vi "Lip_Symmetry_new.vi"(0 "Image in":T3(plugin-control), 1 "Lip Outer Perpendicular lines":T2(array[cluster]), 2 "Box Edge Information":T1, 5 "error in (no error)":errorcluster, 6 "Calibrated Image":T3) -> (14 "Lip symmetry":dbl, 19 "error out":errorcluster)   [LabVIEW 2019, in "Algorithm.lvclass"]
uses:
  FrameworkOverrides/Algorithm.lvclass
  <vilib>/vision/NI_Vision_Development_Module.lvlib
  <vilib>/vision/Image Controls.llb/IMAQ Image.ctl
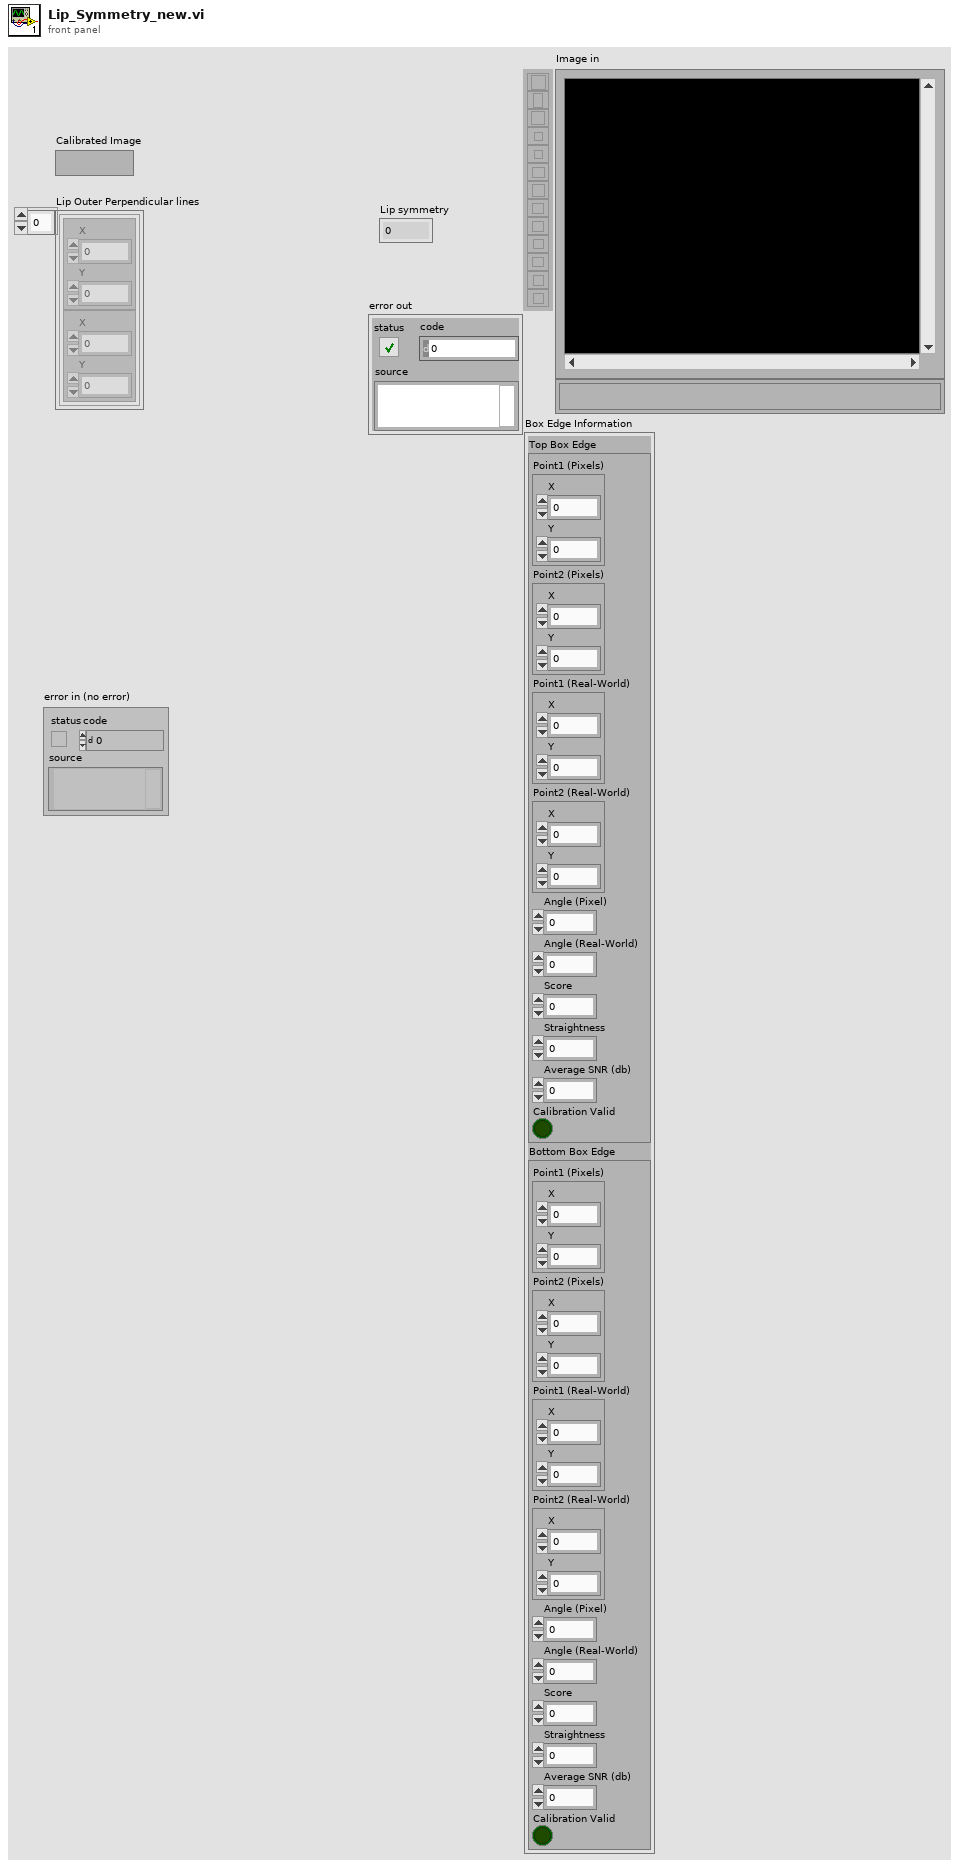
[diagram p1: front panel]
types:
  T1 = cluster{"Top Box Edge":cluster{"Point1 (Pixels)":cluster{"X":sgl, "Y":sgl}, "Point2 (Pixels)":cluster{"X":sgl, "Y":sgl}, "Point1 (Real-World)":cluster{"X":sgl, "Y":sgl}, "Point2 (Real-World)":cluster{"X":sgl, "Y":sgl}, "Angle (Pixel)":dbl, "Angle (Real-World)":dbl, "Score":dbl, "Straightness":dbl, "Average SNR (db)":dbl, "Calibration Valid":bool}, "Bottom Box Edge":cluster{"Point1 (Pixels)":cluster{"X":sgl, "Y":sgl}, "Point2 (Pixels)":cluster{"X":sgl, "Y":sgl}, "Point1 (Real-World)":cluster{"X":sgl, "Y":sgl}, "Point2 (Real-World)":cluster{"X":sgl, "Y":sgl}, "Angle (Pixel)":dbl, "Angle (Real-World)":dbl, "Score":dbl, "Straightness":dbl, "Average SNR (db)":dbl, "Calibration Valid":bool}}
  T2 = cluster{cluster{"X":sgl, "Y":sgl}, cluster{"X":sgl, "Y":sgl}}[]
  T3 = typedef "IMAQ Image.ctl" = refnum<image>
  T4 = cluster{"Point1 (Pixels)":cluster{"X":sgl, "Y":sgl}, "Point2 (Pixels)":cluster{"X":sgl, "Y":sgl}, "Point1 (Real-World)":cluster{"X":sgl, "Y":sgl}, "Point2 (Real-World)":cluster{"X":sgl, "Y":sgl}, "Angle (Pixel)":dbl, "Angle (Real-World)":dbl, "Score":dbl, "Straightness":dbl, "Average SNR (db)":dbl, "Calibration Valid":bool}
  T5 = cluster{"Point1 (Pixels)":cluster{"X":sgl, "Y":sgl}, "Point2 (Pixels)":cluster{"X":sgl, "Y":sgl}}
  T6 = cluster{cluster{"X":sgl, "Y":sgl}, cluster{"X":sgl, "Y":sgl}}
  T7 = cluster{"Point 1":cluster{"X":sgl, "Y":sgl}, "Point 2":cluster{"X":sgl, "Y":sgl}}
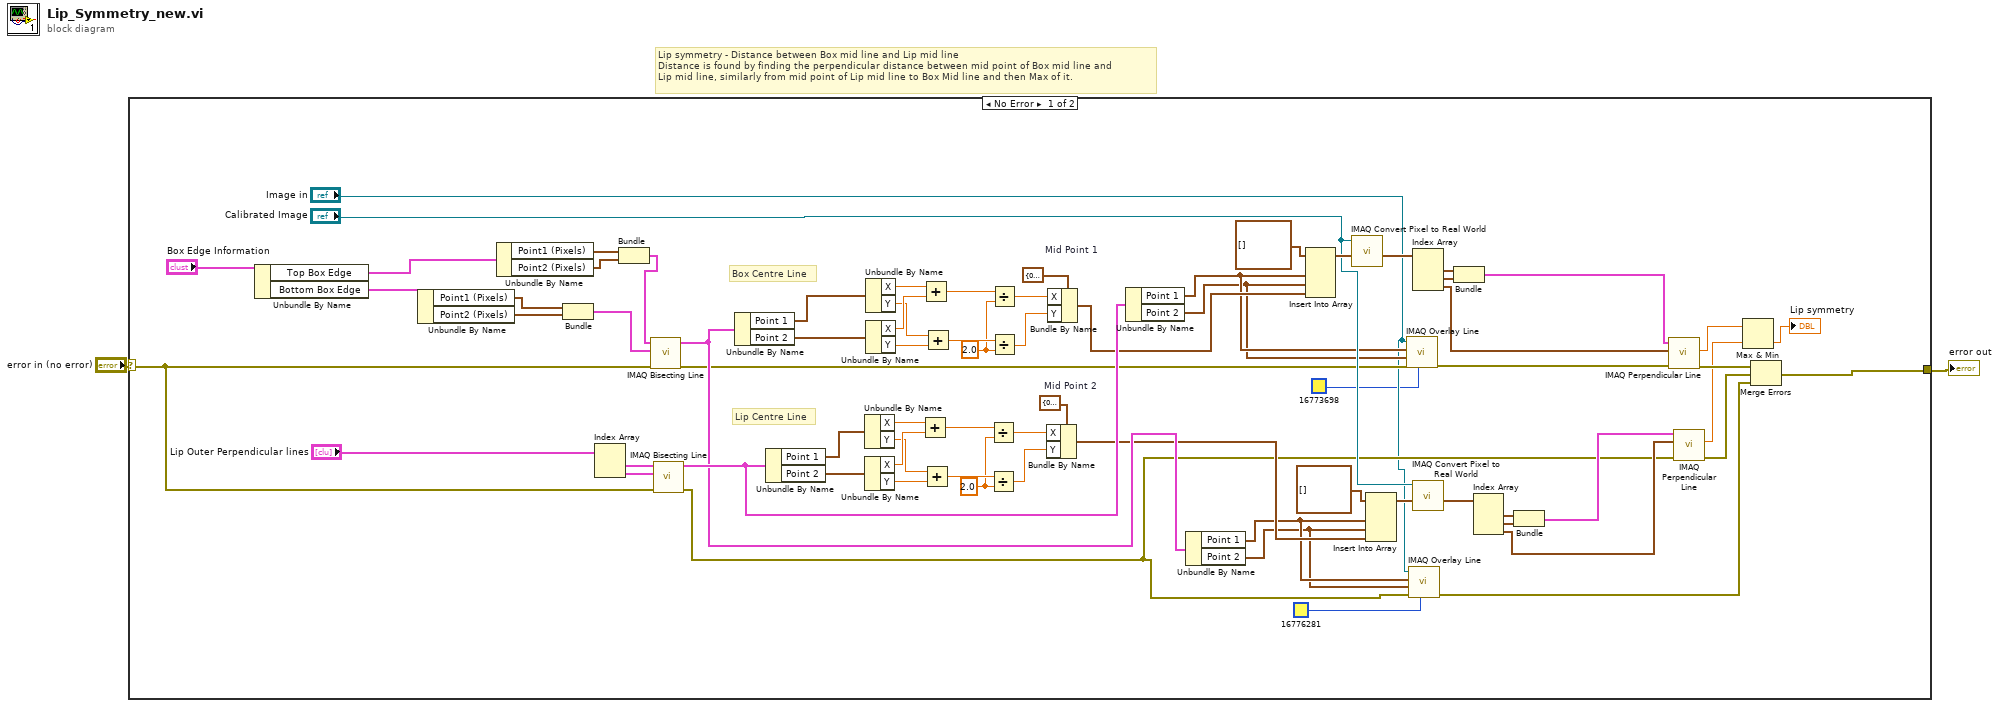
[diagram p0: block diagram]
diagram:
  # "Lip symmetry - Distance between Box mid line and Lip mid line\nDistance is found by finding the perpendicular distance between mid point of Box mid line and\nLip mid line, similarly from mid point of Lip mid line to Box Mid line and then Max of it."
  n1 = case shown="No Error" "error in (no error)" {
    selector: "error in (no error)" -> [w4 w76]
    tunnel: [w48 w76] -> w1
    frame No Error {
      w54 = sgl 2.0 ("y")
      w64 = sgl 2.0 ("y")
      # "Lip Centre Line"
      # "Box Centre Line"
      n2 = Unbundle By Name("Box Edge Information") -> ("Top Box Edge"=w12:T4, "Bottom Box Edge"=w11:T4)
      n3 = Unbundle By Name(w11) -> ("Point1 (Pixels)"=w7:cluster{"X":sgl, "Y":sgl}, "Point2 (Pixels)"=w6:cluster{"X":sgl, "Y":sgl})
      n4 = Unbundle By Name(w12) -> ("Point1 (Pixels)"=w10:cluster{"X":sgl, "Y":sgl}, "Point2 (Pixels)"=w9:cluster{"X":sgl, "Y":sgl})
      n5 = Bundle("Point1 (Pixels)"=w7, "Point2 (Pixels)"=w6) -> (w5:T5)  [unwired: 1 in]
      n6 = Index Array(array="Lip Outer Perpendicular lines") -> (element #1=w74:T6, element #2=w73:T6)  [unwired: 2 in]
      n7 = Bundle("Point1 (Pixels)"=w10, "Point2 (Pixels)"=w9) -> (w8:T5)  [unwired: 1 in]
      n8 = call "IMAQ Bisecting Line"("error in (no error)"=w4, "Line 2"=w5, "Line 1"=w8) -> ("error out"=w19:errorcluster, "Bisecting Line"=w29:T7)  [unwired: 7 in]
      n9 = call "IMAQ Bisecting Line"("error in (no error)"=w4, "Line 2"=w73, "Line 1"=w74) -> ("error out"=w20:errorcluster, "Bisecting Line"=w43:T7)  [unwired: 7 in]
      n10 = Unbundle By Name(w29) -> ("Point 1"=w72:cluster{"X":sgl, "Y":sgl}, "Point 2"=w71:cluster{"X":sgl, "Y":sgl})
      n11 = Unbundle By Name(w43) -> ("Point 1"=w50:cluster{"X":sgl, "Y":sgl}, "Point 2"=w49:cluster{"X":sgl, "Y":sgl})
      n12 = Unbundle By Name(w50) -> ("X"=w60:sgl, "Y"=w58:sgl)
      n13 = Unbundle By Name(w49) -> ("X"=w59:sgl, "Y"=w57:sgl)
      n14 = Unbundle By Name(w72) -> ("X"=w70:sgl, "Y"=w68:sgl)
      n15 = Unbundle By Name(w71) -> ("X"=w69:sgl, "Y"=w67:sgl)
      n16 = Add(x=w60, y=w59) -> (x+y=w56:sgl)
      n17 = Add(x=w70, y=w69) -> (x+y=w66:sgl)
      n18 = Add(x=w58, y=w57) -> (x+y=w55:sgl)
      n19 = Add(x=w68, y=w67) -> (x+y=w65:sgl)
      n20 = Divide(x=w56, y=w54) -> (x/y=w52:sgl)
      n21 = Divide(x=w55, y=w54) -> (x/y=w51:sgl)
      n22 = Divide(x=w66, y=w64) -> (x/y=w62:sgl)
      n23 = Divide(x=w65, y=w64) -> (x/y=w61:sgl)
      n24 = Bundle By Name "Mid Point 2"(cluster=cluster{"X":sgl, "Y":sgl} {"X"=0.0, "Y"=0.0} ("Point 1"), "X"=w52, "Y"=w51) -> (w27:cluster{"X":sgl, "Y":sgl})
      n25 = Bundle By Name "Mid Point 1"(cluster=cluster{"X":sgl, "Y":sgl} {"X"=0.0, "Y"=0.0} ("Point 1"), "X"=w62, "Y"=w61) -> (w36:cluster{"X":sgl, "Y":sgl})
      n26 = Unbundle By Name(w43) -> ("Point 1"=w24:cluster{"X":sgl, "Y":sgl}, "Point 2"=w23:cluster{"X":sgl, "Y":sgl})
      n27 = Unbundle By Name(w29) -> ("Point 1"=w22:cluster{"X":sgl, "Y":sgl}, "Point 2"=w21:cluster{"X":sgl, "Y":sgl})
      n28 = Insert Into Array(array=cluster{"X":sgl, "Y":sgl}[] [] ("appended array"), new element #1=w24, new element #2=w23, new element #3=w36) -> (w41:cluster{"X":sgl, "Y":sgl}[])  [unwired: 1 in]
      n29 = call "IMAQ Convert Pixel to Real World"("Array of Pixel Coordinates"=w41, "Calibrated Image"="Calibrated Image") -> ("Array of Real World Coordinates"=w40:cluster{"X":sgl, "Y":sgl}[])  [unwired: 4 in, 5 out]
      n30 = Insert Into Array(array=cluster{"X":sgl, "Y":sgl}[] [] ("appended array"), new element #1=w22, new element #2=w21, new element #3=w27) -> (w33:cluster{"X":sgl, "Y":sgl}[])  [unwired: 1 in]
      n31 = call "IMAQ Overlay Line"("Color"=u32 16773698, "error in (no error)"=w19, "End Point"=w23, "Start Point"=w24, "Image"="Image in") -> ("error out"=w18:errorcluster)  [unwired: 5 in, 1 out]
      n32 = call "IMAQ Overlay Line"("Color"=u32 16776281, "error in (no error)"=w20, "End Point"=w21, "Start Point"=w22, "Image"="Image in") -> ("error out"=w17:errorcluster)  [unwired: 5 in, 1 out]
      n33 = Index Array(array=w40) -> (element #1=w39:cluster{"X":sgl, "Y":sgl}, element #2=w38:cluster{"X":sgl, "Y":sgl}, element #3=w35:cluster{"X":sgl, "Y":sgl})  [unwired: 3 in]
      n34 = call "IMAQ Convert Pixel to Real World"("Array of Pixel Coordinates"=w33, "Calibrated Image"="Calibrated Image") -> ("Array of Real World Coordinates"=w32:cluster{"X":sgl, "Y":sgl}[])  [unwired: 4 in, 5 out]
      n35 = Bundle(w39, w38) -> (w37:T6)  [unwired: 1 in]
      n36 = Index Array(array=w32) -> (element #1=w31:cluster{"X":sgl, "Y":sgl}, element #2=w30:cluster{"X":sgl, "Y":sgl}, element #3=w26:cluster{"X":sgl, "Y":sgl})  [unwired: 3 in]
      n37 = Bundle(w31, w30) -> (w28:T6)  [unwired: 1 in]
      n38 = call "IMAQ Perpendicular Line"("error in (no error)"=w18, "Point"=w35, "Line"=w37) -> ("error out"=w47:errorcluster, "Distance"=w46:dbl)  [unwired: 6 in, 1 out]
      n39 = call "IMAQ Perpendicular Line"("error in (no error)"=w20, "Point"=w26, "Line"=w28) -> ("error out"=w44:errorcluster, "Distance"=w45:dbl)  [unwired: 6 in, 1 out]
      n40 = Max & Min(x=w46, y=w45) -> (min(x,y)=→"Lip symmetry":dbl)  [unwired: 1 out]
      n41 = Merge Errors(w47, w44, w17) -> (w48:errorcluster)
    }
    frame Error {
    }
  }
  "error out" <- w1
